vi "dfd_Extract Content Between Tags.vi"(10 "element":string, 11 "xml string with tag":string) -> (2 "remaining string":string, 3 "content":string)   [LabVIEW 2017, in "NI_DigFilter_Process.lvlib"]
uses:
  <vilib>/addons/Digital Filter Design/NI_DigFilter_Process.lvlib
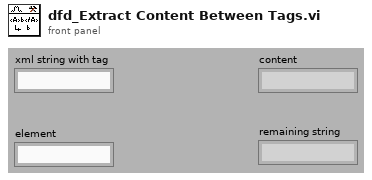
[diagram p1: front panel]
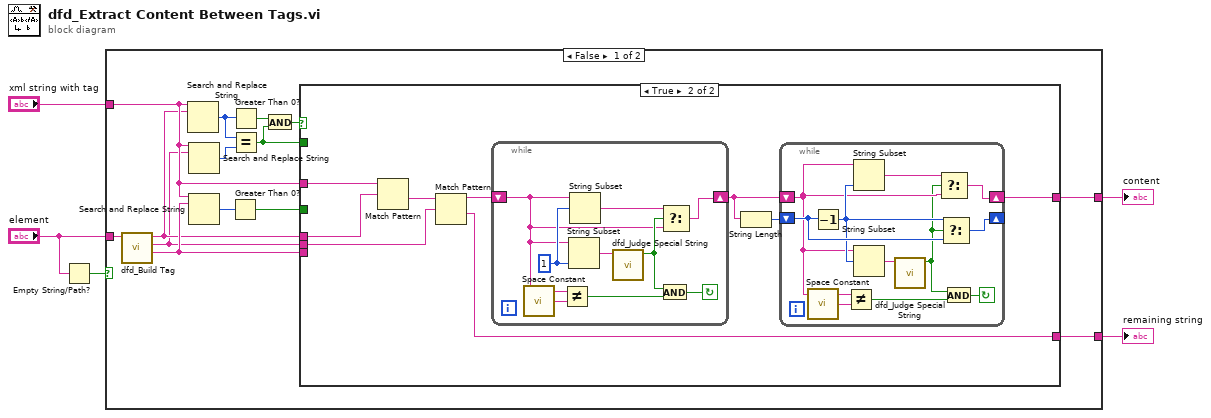
[diagram p0: block diagram]
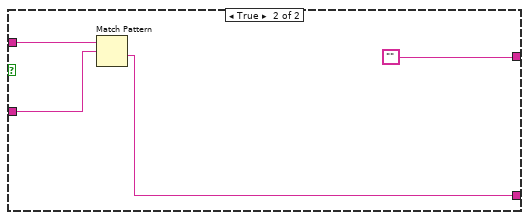
[diagram p4: hidden frame]
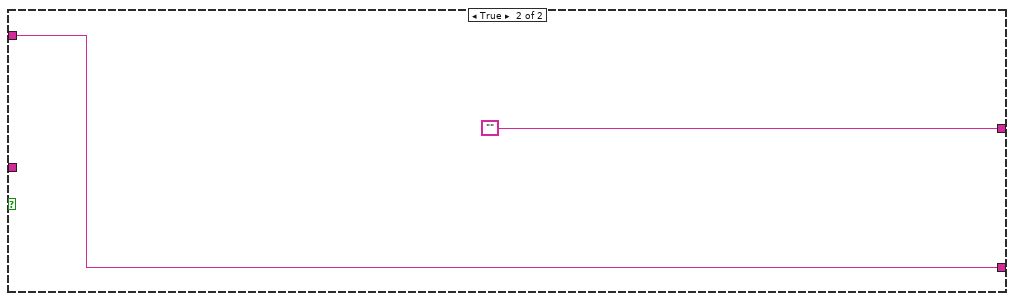
[diagram p5: hidden frame]
diagram:
  n1 = Empty String/Path?(string/path="element") -> (empty?=w1:bool)
  n2 = case shown="False" w1 {
    tunnel: "element" -> [w19 _]
    tunnel: "xml string with tag" -> [w13 w66]
    tunnel: [w18 ""] -> w4
    tunnel: [w17 w66] -> w3
    frame False {
      n3 = call <vilib>:"dfd_Build Tag.vi"("element name"=w19) -> ("empty tag"=w14:string, "end tag"=w11:string, "start tag"=w12:string)  [unwired: 8 out]
      n4 = Search and Replace String(input string=w13, search string=w12) -> (number of replacements=w9:i32)  [unwired: 1 in, 8 out]
      n5 = Search and Replace String(input string=w13, search string=w11) -> (number of replacements=w10:i32)  [unwired: 1 in, 8 out]
      n6 = Search and Replace String(input string=w13, search string=w14) -> (number of replacements=w16:i32)  [unwired: 1 in, 8 out]
      n7 = Greater Than 0?(x=w16) -> (x > 0?=w15:bool)
      n8 = Greater Than 0?(x=w9) -> (x > 0?=w8:bool)
      n9 = Equal?(x=w9, y=w10) -> (x = y?=w6:bool)
      n10 = And(x=w8, y=w6) -> (x .and. y?=w7:bool)
      n11 = case shown="True" w7 {
        tunnel: [w23 w44] -> w18
        tunnel: [w22 w43] -> w17
        tunnel: w15 -> [w21 _]
        tunnel: w14 -> [w24 _]
        tunnel: w13 -> [w25 w42]
        tunnel: w12 -> [_ w37]
        tunnel: w11 -> [_ w36]
        tunnel: w6 -> [w20 _]
        frame False {
          n12 = case shown="True" w20 {
            tunnel: w25 -> [_ w30]
            tunnel: w24 -> [_ w29]
            tunnel: [_ w28] -> w23
            tunnel: [_ w27] -> w22
            tunnel: w21 -> [_ w26]
            frame False {
            }
            frame True {
              n13 = case shown="False" w26 {
                tunnel: [_ ""] -> w28
                tunnel: [w31 w33] -> w27
                tunnel: w30 -> [w31 w35]
                tunnel: w29 -> [_ w34]
                frame False {
                }
                frame True {
                  n14 = Match Pattern(string=w35, regular expression=w34) -> (after substring=w33:string)  [unwired: 4 out]
                }
              }
            }
          }
        }
        frame True {
          n15 = Match Pattern(string=w42, regular expression=w37) -> (after substring=w38:string)  [unwired: 4 out]
          n16 = Match Pattern(string=w38, regular expression=w36) -> (before substring=w41:string, after substring=w43:string)  [unwired: 3 out]
          n17 = while {
            shift-right: [w62] -> w39
            shift-left: w41 -> [w56]
            stop <- w59 continue-if-true
            w64 = 1 ("length (rest)")
            n18 = call <vilib>:"Space Constant.vi"() -> ("String"=w57:string)
            n19 = Not Equal?(x=w56, y=w57) -> (x != y?=w58:bool)
            n20 = String Subset(string=w56, length (rest)=w64) -> (substring=w61:string)  [unwired: 1 out]
            n21 = String Subset(string=w56, offset (0)=w64) -> (substring=w63:string)  [unwired: 1 out]
            n22 = call <vilib>:"dfd_Judge Special String.vi"("string"=w61) -> ("space ?"=w60:bool)  [unwired: 10 out]
            n23 = And(x=w60, y=w58) -> (x .and. y?=w59:bool)
            n24 = Select(t=w63, s=w60, f=w56) -> (s? t:f=w62:string)
          }
          n25 = String Length(string=w39) -> (length=w40:i32)
          n26 = while {
            shift-right: [w53] -> _
            shift-left: w40 -> [w51]
            shift-right: [w54] -> w44
            shift-left: w39 -> [w47]
            stop <- w45 continue-if-true
            n27 = call <vilib>:"Space Constant.vi"() -> ("String"=w49:string)
            n28 = Decrement(x=w51) -> (x-1=w50:i32)
            n29 = Not Equal?(x=w47, y=w49) -> (x != y?=w48:bool)
            n30 = String Subset(string=w47, length (rest)=w50) -> (substring=w55:string)  [unwired: 1 out]
            n31 = String Subset(string=w47, offset (0)=w50) -> (substring=w52:string)  [unwired: 1 out]
            n32 = call <vilib>:"dfd_Judge Special String.vi"("string"=w52) -> ("space ?"=w46:bool)  [unwired: 10 out]
            n33 = Select(t=w55, s=w46, f=w47) -> (s? t:f=w54:string)
            n34 = Select(t=w50, s=w46, f=w51) -> (s? t:f=w53:i32)
            n35 = And(x=w46, y=w48) -> (x .and. y?=w45:bool)
          }
        }
      }
    }
    frame True {
    }
  }
  "content" <- w4
  "remaining string" <- w3
